vi "generate waveforms.vi"(10 "Number of Samples":i32=128) -> (1 "Y SCan Waveform":waveform(dbl), 2 "X Scan Waveform":waveform(dbl), 4 "Y Scan Raw":dbl[](array[numeric]), 5 "X Scan Raw":dbl[](array[numeric]))   [LabVIEW 2012]
uses:
  <vilib>/Analysis/NI_AALBase.lvlib
  <vilib>/Analysis/1siggen.llb/Ramp Pattern by Samples.vi
panel:
  out "error":i32
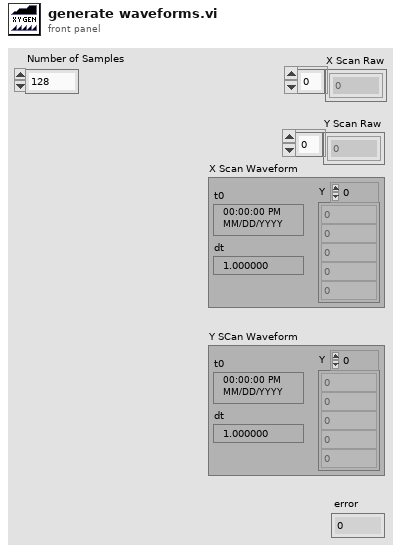
[diagram p1: front panel]
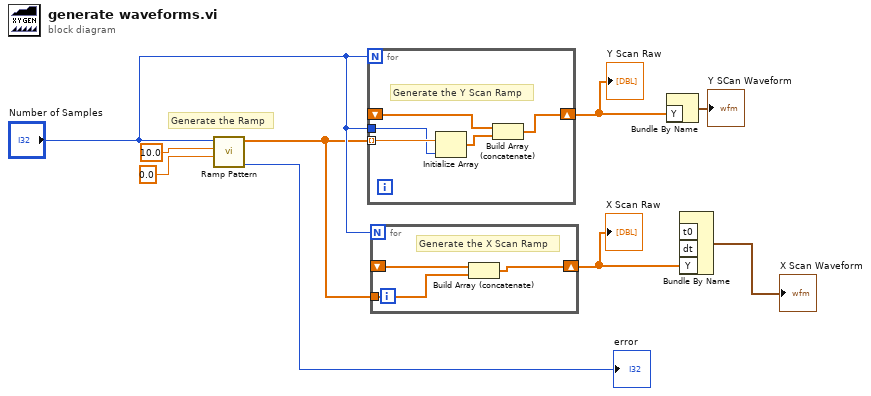
[diagram p0: block diagram]
diagram:
  # "Generate the Ramp"
  n1 = call-poly <vilib>:"Ramp Pattern.vi"("start"=0.0, "end"=10.0, "samples"="Number of Samples") -> ("error"=→"error":i32, "Ramp Pattern"=w6:dbl[])  [unwired: 7 in]
  n2 = for {
    N: "Number of Samples" -> [_]
    tunnel: w6 -> [w14] mode=indexing
    tunnel: "Number of Samples" -> [w13]
    shift-right: [w11] -> w3
    shift-left: _ -> [w10]
    # "Generate the Y Scan Ramp"
    n3 = Initialize Array(w14, w13) -> (w12:dbl[])
    n4 = Build Array (concatenate)(w10, w12) -> (w11:dbl[])
  }
  "Y Scan Raw" <- w3
  n5 = for {
    N: "Number of Samples" -> [_]
    tunnel: w6 -> [w17]
    shift-right: [w16] -> w4
    shift-left: _ -> [w15]
    # "Generate the X Scan Ramp"
    n6 = Build Array (concatenate)(w15, w17) -> (w16:dbl[])
  }
  "X Scan Raw" <- w4
  n7 = Bundle By Name("Y"=w3) -> (→"Y SCan Waveform":waveform(dbl))  [unwired: 1 in]
  n8 = Bundle By Name("Y"=w4) -> (→"X Scan Waveform":waveform(dbl))  [unwired: 3 in]
